vi "WLAN - TV - RW - UTIL - TestVectors_11N.vi"(0 "TV_IQComposite_11N":T2={"Standard"=3, "80211n PLCP Frame Format"=[0], "FEC Coding Type"=[0], "Guard Interval (s)"=[0.0], "OFDM Advanced Controls"={"OFDM Auto Compute Acquisition Length Enabled"=0, "OFDM Maximum Symbols Used"=0, "OFDM Time Tracking Enabled"=0, "OFDM Channel Tracking Enabled"=0, "OFDM Amplitude Tracking Enabled"=1, "OFDM CFO Estimation Method"=0, "OFDM Phase Tracking Method"=0, "OFDM Header Detection Enabled"=0, "OFDM MAC FCS Check Enabled"=0, "#Avg"=10, "#Iterations"=10}, "Generation Parameters"=[], "Measurement Enabled"=FALSE, "#Packets"=0} {"Generation Parameters"."Center Frequency(Hz)" format="%#_6p"; "Generation Parameters"."Generation Parameters"."Channel Bandwidth(Hz)" items=["5M"=5000000.0, "10M"=10000000.0, "20M"=20000000.0, "40M"=40000000.0, "80M"=80000000.0, "160M"=160000000.0]; "OFDM Advanced Controls"."OFDM Phase Tracking Method" items=["Standard", "Instantaneous", "None", "Standard with Cubic Spline Fit"]; "OFDM Advanced Controls"."OFDM CFO Estimation Method" items=["Preamble Only", "Preamble and Data"]; "OFDM Advanced Controls"."OFDM Channel Tracking Enabled" items=["False", "True"]; "OFDM Advanced Controls"."OFDM Amplitude Tracking Enabled" items=["False", "True"]; "OFDM Advanced Controls"."OFDM Time Tracking Enabled" items=["True"=1, "False"=0]; "OFDM Advanced Controls"."OFDM Auto Compute Acquisition Length Enabled" items=["False", "True"]; "OFDM Advanced Controls"."OFDM MAC FCS Check Enabled" items=["False", "True"]; "OFDM Advanced Controls"."OFDM Header Detection Enabled" items=["False", "True"]; "FEC Coding Type" items=["BCC", "LDPC"]; "80211n PLCP Frame Format" items=["Mixed Format", "Greenfield Format"]; "Standard" items=["80211A/G/J/P OFDM", "80211B/G DSSS", "80211G DSSSOFDM", "80211N MIMOOFDM", "80211AC MIMOOFDM"]}, 1 "11n_Meas_Config":path, 3 "TV_802_11n":path, 7 "TV Paramaters":T1) -> ()   [LabVIEW 2011]
uses:
  Includes/WLAN - TV - RW - INC - TV_IQComposite_11N.ctl
  Includes/WLAN - TV - RW - INC - TV_OFDM Demod.ctl
  Includes/WLAN - TV - RW - INC - TV_Parameters.ctl
  Includes/WLAN - TV - RW - INC - Tx_Meas_Settings_OFDM_String.ctl
  <vilib>/Utility/file.llb/Write To Spreadsheet File (string).vi
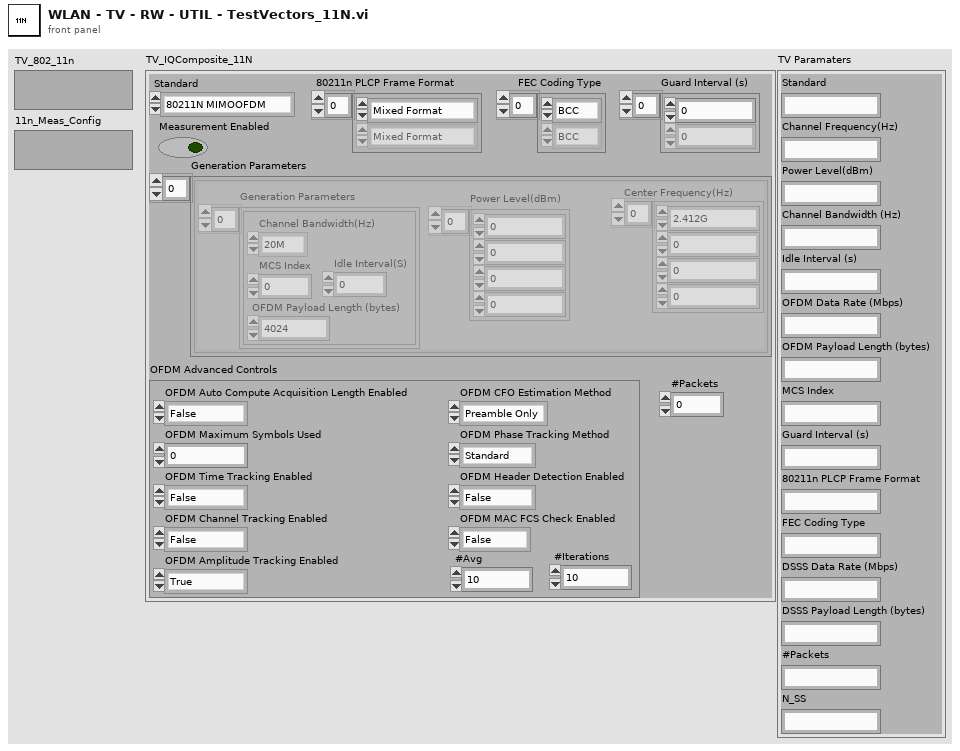
[diagram p1: front panel]
types:
  T1 = typedef "WLAN - TV - RW - INC - TV_Parameters.ctl" = cluster{"Standard ":string, "Channel Frequency(Hz)":string, "Power Level(dBm)":string, "Channel Bandwidth (Hz)":string, "Idle Interval (s)":string, "OFDM Data Rate (Mbps)":string, "OFDM Payload Length (bytes)":string, "MCS Index":string, "Guard Interval (s)":string, "80211n PLCP Frame Format":string, "FEC Coding Type":string, "DSSS Data Rate (Mbps)":string, "DSSS Payload Length (bytes)":string, "#Packets":string, "N_SS":string}
  T2 = typedef "WLAN - TV - RW - INC - TV_IQComposite_11N.ctl" = cluster{"Standard":i32, "80211n PLCP Frame Format":i32[], "FEC Coding Type":i32[], "Guard Interval (s)":dbl[], "OFDM Advanced Controls":T3, "Generation Parameters":cluster{"Generation Parameters":cluster{"Channel Bandwidth(Hz)":dbl, "MCS Index":i32, "OFDM Payload Length (bytes)":i32, "Idle Interval(S)":dbl}[], "Center Frequency(Hz)":dbl[], "Power Level(dBm)":dbl[]}[], "Measurement Enabled":bool, "#Packets":i32}
  T3 = typedef "WLAN - TV - RW - INC - TV_OFDM Demod.ctl" = cluster{"OFDM Auto Compute Acquisition Length Enabled":i32, "OFDM Maximum Symbols Used":i32, "OFDM Time Tracking Enabled":i32, "OFDM Channel Tracking Enabled":i32, "OFDM Amplitude Tracking Enabled":i32, "OFDM CFO Estimation Method":i32, "OFDM Phase Tracking Method":i32, "OFDM Header Detection Enabled":i32, "OFDM MAC FCS Check Enabled":i32, "#Avg":i32, "#Iterations":i32}
  T4 = typedef "WLAN - TV - RW - INC - Tx_Meas_Settings_OFDM_String.ctl" = cluster{"OFDM Auto Compute Acquisition Length Enabled":string, "OFDM Maximum Symbols Used":string, "OFDM Time Tracking Enabled":string, "OFDM Channel Tracking Enabled":string, "OFDM Amplitude Tracking Enabled":string, "OFDM CFO Estimation Method":string, "OFDM Phase Tracking Method":string, "OFDM Header Detection Enabled":string, "OFDM MAC FCS Check Enabled":string, "#Avg":string, "#Iterations":string}
  T5 = cluster{"Generation Parameters":cluster{"Channel Bandwidth(Hz)":dbl, "MCS Index":i32, "OFDM Payload Length (bytes)":i32, "Idle Interval(S)":dbl}[], "Center Frequency(Hz)":dbl[], "Power Level(dBm)":dbl[]}[]
  T6 = cluster{"Channel Bandwidth(Hz)":dbl, "MCS Index":i32, "OFDM Payload Length (bytes)":i32, "Idle Interval(S)":dbl}[]
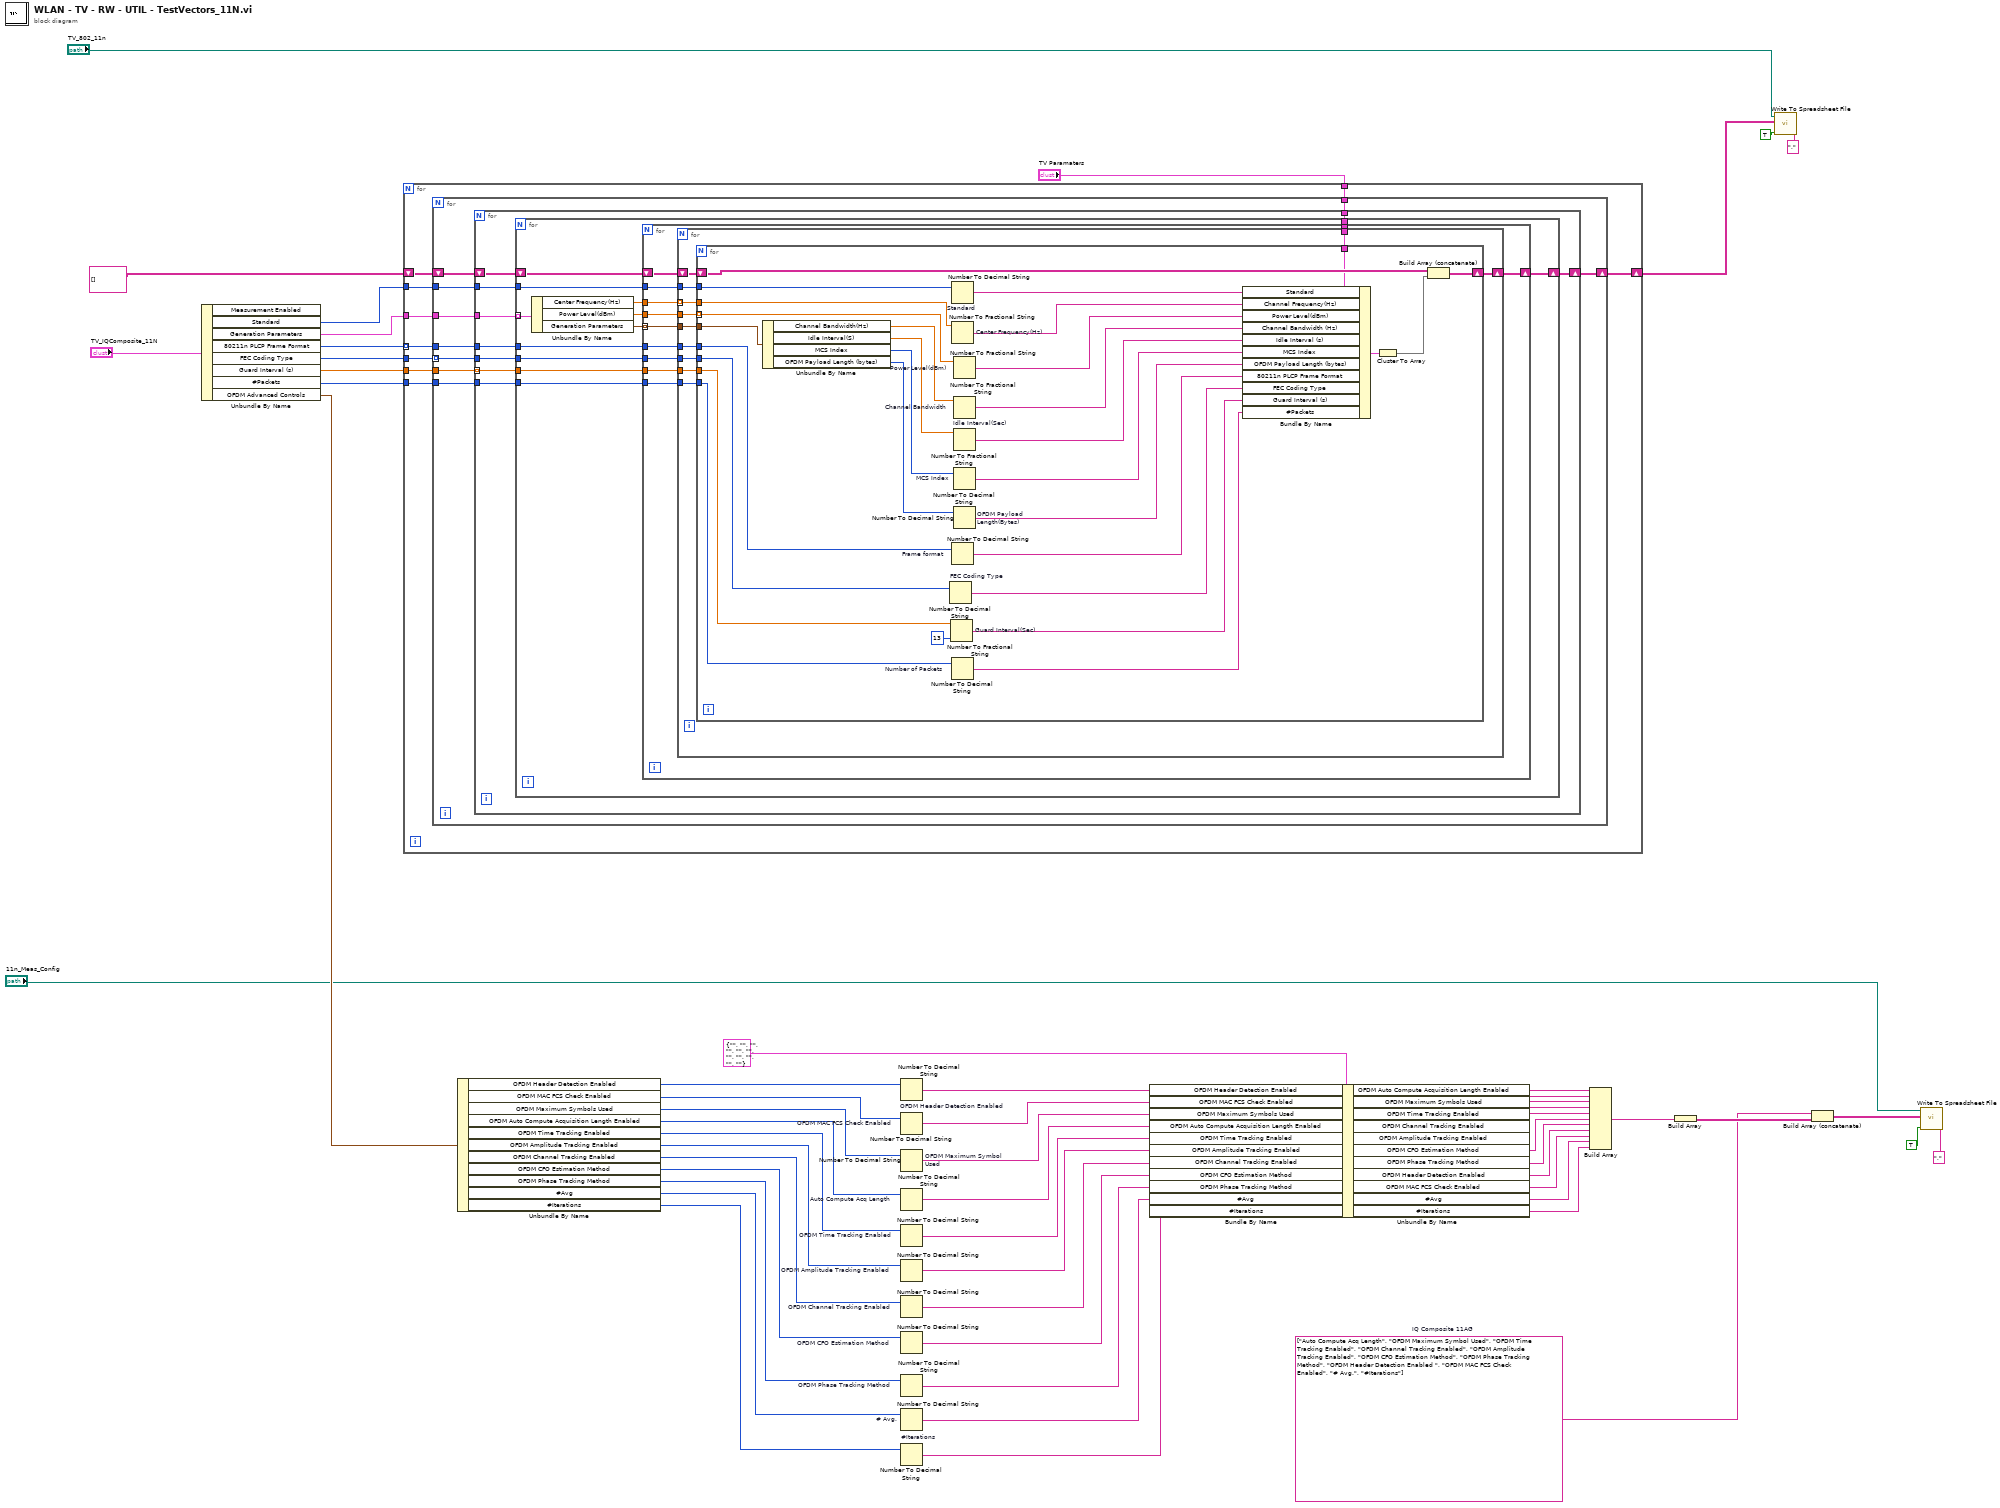
[diagram p0: block diagram]
diagram:
  w2 = string[] ["Auto Compute Acq Length", "OFDM Maximum Symbol Used", "OFDM Time Tracking Enabled", "OFDM Channel Tracking Enabled", "OFDM Amplitude Tracking Enabled", "OFDM CFO Estimation Method", "OFDM Phase Tracking Method", "OFDM Header Detection Enabled ", "OFDM MAC FCS Check Enabled", "# Avg.", "#Iterations"]  # IQ Composite 11AG
  n1 = Unbundle By Name("TV_IQComposite_11N") -> ("Standard"=w52:i32, "Generation Parameters"=w47:T5, "80211n PLCP Frame Format"=w48:i32[], "FEC Coding Type"=w56:i32[], "Guard Interval (s)"=w55:dbl[], "#Packets"=w46:i32, "OFDM Advanced Controls"=w5:T3)  [unwired: 1 out]
  n2 = for {
    tunnel: w48 -> [w65] mode=indexing
    tunnel: w56 -> [w64]
    tunnel: w55 -> [w63]
    tunnel: w52 -> [w62]
    tunnel: "TV Paramaters" -> [w61]
    shift-right: [w60] -> w1
    shift-left: string[][] [] ("appended array") -> [w59]
    tunnel: w47 -> [w58]
    tunnel: w46 -> [w57]
    n3 = for {
      tunnel: w65 -> [w74]
      tunnel: w64 -> [w73] mode=indexing
      tunnel: w63 -> [w72]
      tunnel: w62 -> [w71]
      tunnel: w61 -> [w70]
      shift-right: [w69] -> w60
      shift-left: w59 -> [w68]
      tunnel: w58 -> [w67]
      tunnel: w57 -> [w66]
      n4 = for {
        tunnel: w74 -> [w83]
        tunnel: w73 -> [w82]
        tunnel: w72 -> [w81] mode=indexing
        tunnel: w71 -> [w80]
        tunnel: w70 -> [w79]
        shift-right: [w78] -> w69
        shift-left: w68 -> [w77]
        tunnel: w67 -> [w76]
        tunnel: w66 -> [w75]
        n5 = for {
          tunnel: w83 -> [w87]
          tunnel: w82 -> [w86]
          tunnel: w81 -> [w85]
          tunnel: w80 -> [w95]
          tunnel: w79 -> [w94]
          shift-right: [w93] -> w78
          shift-left: w77 -> [w89]
          tunnel: w76 -> [w88] mode=indexing
          tunnel: w75 -> [w84]
          n6 = Unbundle By Name(w88) -> ("Center Frequency(Hz)"=w91:dbl[], "Power Level(dBm)"=w90:dbl[], "Generation Parameters"=w92:T6)
          n7 = for {
            tunnel: w95 -> [w106]
            tunnel: w94 -> [w105]
            tunnel: w92 -> [w103] mode=indexing
            tunnel: w91 -> [w102]
            tunnel: w90 -> [w101]
            shift-right: [w104] -> w93
            shift-left: w89 -> [w100]
            tunnel: w87 -> [w99]
            tunnel: w86 -> [w98]
            tunnel: w85 -> [w97]
            tunnel: w84 -> [w96]
            n8 = for {
              shift-right: [w116] -> w104
              shift-left: w100 -> [w117]
              tunnel: w106 -> [w115]
              tunnel: w105 -> [w114]
              tunnel: w103 -> [w113]
              tunnel: w102 -> [w112] mode=indexing
              tunnel: w101 -> [w111]
              tunnel: w99 -> [w110]
              tunnel: w98 -> [w109]
              tunnel: w97 -> [w108]
              tunnel: w96 -> [w107]
              n9 = for {
                shift-right: [w146] -> w116
                shift-left: w117 -> [w145]
                tunnel: w115 -> [w144]
                tunnel: w114 -> [w143]
                tunnel: w113 -> [w130]
                tunnel: w112 -> [w131]
                tunnel: w111 -> [w132] mode=indexing
                tunnel: w110 -> [w125]
                tunnel: w109 -> [w124]
                tunnel: w108 -> [w123]
                tunnel: w107 -> [w122]
                n10 = Unbundle By Name(w130) -> ("Channel Bandwidth(Hz)"=w126:dbl, "Idle Interval(S)"=w127:dbl, "MCS Index"=w128:i32, "OFDM Payload Length (bytes)"=w129:i32)
                n11 = Number To Decimal String "FEC Coding Type"(number=w124) -> (decimal integer string=w133:string)  [unwired: 1 in]
                n12 = Number To Fractional String "Guard Interval(Sec)"(number=w123, precision (6)=i16 13) -> (F-format string=w134:string)  [unwired: 2 in]
                n13 = Number To Decimal String "Frame format"(number=w125) -> (decimal integer string=w135:string)  [unwired: 1 in]
                n14 = Number To Decimal String "Number of Packets"(number=w122) -> (decimal integer string=w121:string)  [unwired: 1 in]
                n15 = Number To Decimal String "Standard"(number=w144) -> (decimal integer string=w136:string)  [unwired: 1 in]
                n16 = Number To Fractional String "Center Frequency(Hz)"(number=w131) -> (F-format string=w137:string)  [unwired: 3 in]
                n17 = Number To Fractional String "Power Level(dBm)"(number=w132) -> (F-format string=w138:string)  [unwired: 3 in]
                n18 = Number To Fractional String "Channel Bandwidth"(number=w126) -> (F-format string=w139:string)  [unwired: 3 in]
                n19 = Number To Fractional String "Idle Interval(Sec)"(number=w127) -> (F-format string=w140:string)  [unwired: 3 in]
                n20 = Number To Decimal String "MCS Index"(number=w128) -> (decimal integer string=w141:string)  [unwired: 1 in]
                n21 = Number To Decimal String "OFDM Payload Length(Bytes)"(number=w129) -> (decimal integer string=w142:string)  [unwired: 1 in]
                n22 = Bundle By Name(cluster=w143, "Standard"=w136, "Channel Frequency(Hz)"=w137, "Power Level(dBm)"=w138, "Channel Bandwidth (Hz)"=w139, "Idle Interval (s)"=w140, "MCS Index"=w141, "OFDM Payload Length (bytes)"=w142, "80211n PLCP Frame Format"=w135, "FEC Coding Type"=w133, "Guard Interval (s)"=w134, "#Packets"=w121) -> (w119:T1)
                n23 = Cluster To Array(cluster=w119) -> (array=w118:string[])
                n24 = Build Array (concatenate)(w145, w118) -> (w146:string[][])
              }
            }
          }
        }
      }
    }
  }
  n25 = Unbundle By Name(w5) -> ("OFDM Header Detection Enabled"=w35:i32, "OFDM MAC FCS Check Enabled"=w36:i32, "OFDM Maximum Symbols Used"=w37:i32, "OFDM Auto Compute Acquisition Length Enabled"=w38:i32, "OFDM Time Tracking Enabled"=w39:i32, "OFDM Amplitude Tracking Enabled"=w40:i32, "OFDM Channel Tracking Enabled"=w41:i32, "OFDM CFO Estimation Method"=w42:i32, "OFDM Phase Tracking Method"=w43:i32, "#Avg"=w44:i32, "#Iterations"=w45:i32)
  n26 = Number To Decimal String "OFDM Header Detection Enabled"(number=w35) -> (decimal integer string=w33:string)  [unwired: 1 in]
  n27 = Number To Decimal String "OFDM MAC FCS Check Enabled"(number=w36) -> (decimal integer string=w32:string)  [unwired: 1 in]
  n28 = Number To Decimal String "OFDM Maximum Symbol Used"(number=w37) -> (decimal integer string=w31:string)  [unwired: 1 in]
  n29 = Number To Decimal String "Auto Compute Acq Length"(number=w38) -> (decimal integer string=w30:string)  [unwired: 1 in]
  n30 = Number To Decimal String "OFDM Time Tracking Enabled"(number=w39) -> (decimal integer string=w29:string)  [unwired: 1 in]
  n31 = Number To Decimal String "OFDM Amplitude Tracking Enabled"(number=w40) -> (decimal integer string=w28:string)  [unwired: 1 in]
  n32 = Number To Decimal String "OFDM Channel Tracking Enabled"(number=w41) -> (decimal integer string=w23:string)  [unwired: 1 in]
  n33 = Number To Decimal String "OFDM CFO Estimation Method"(number=w42) -> (decimal integer string=w24:string)  [unwired: 1 in]
  n34 = Number To Decimal String "OFDM Phase Tracking Method"(number=w43) -> (decimal integer string=w25:string)  [unwired: 1 in]
  n35 = Number To Decimal String "# Avg."(number=w44) -> (decimal integer string=w26:string)  [unwired: 1 in]
  n36 = Number To Decimal String "#Iterations"(number=w45) -> (decimal integer string=w27:string)  [unwired: 1 in]
  n37 = Bundle By Name(cluster=T4 {"OFDM Auto Compute Acquisition Length Enabled"="", "OFDM Maximum Symbols Used"="", "OFDM Time Tracking Enabled"="", "OFDM Channel Tracking Enabled"="", "OFDM Amplitude Tracking Enabled"="", "OFDM CFO Estimation Method"="", "OFDM Phase Tracking Method"="", "OFDM Header Detection Enabled"="", "OFDM MAC FCS Check Enabled"="", "#Avg"="", "#Iterations"=""} ("OFDM Measurement Settings"), "OFDM Header Detection Enabled"=w33, "OFDM MAC FCS Check Enabled"=w32, "OFDM Maximum Symbols Used"=w31, "OFDM Auto Compute Acquisition Length Enabled"=w30, "OFDM Time Tracking Enabled"=w29, "OFDM Amplitude Tracking Enabled"=w28, "OFDM Channel Tracking Enabled"=w23, "OFDM CFO Estimation Method"=w24, "OFDM Phase Tracking Method"=w25, "#Avg"=w26, "#Iterations"=w27) -> (w20:T4)
  n38 = Unbundle By Name(w20) -> ("OFDM Auto Compute Acquisition Length Enabled"=w19:string, "OFDM Maximum Symbols Used"=w18:string, "OFDM Time Tracking Enabled"=w17:string, "OFDM Channel Tracking Enabled"=w16:string, "OFDM Amplitude Tracking Enabled"=w15:string, "OFDM CFO Estimation Method"=w14:string, "OFDM Phase Tracking Method"=w13:string, "OFDM Header Detection Enabled"=w12:string, "OFDM MAC FCS Check Enabled"=w11:string, "#Avg"=w10:string, "#Iterations"=w9:string)
  n39 = Build Array(w19, w18, w17, w16, w15, w14, w13, w12, w11, w10, w9) -> (w8:string[])
  n40 = Build Array(w8) -> (w6:string[][])
  n41 = call-poly <vilib>:"Write To Spreadsheet File.vi"("delimiter (\\t)"="," ("delimiter (\\t)"), "append to file? (new file:F)"=TRUE, "2D data"=w1, "file path (dialog if empty)"="TV_802_11n") -> ()  [unwired: 4 in, 1 out]
  n42 = Build Array (concatenate)(w2, w6) -> (w7:string[][])
  n43 = call-poly <vilib>:"Write To Spreadsheet File.vi"("delimiter (\\t)"="," ("delimiter (\\t)"), "append to file? (new file:F)"=TRUE, "2D data"=w7, "file path (dialog if empty)"="11n_Meas_Config") -> ()  [unwired: 4 in, 1 out]
